vi "与工控机通讯.vi"(10 "values":u16[](array[numeric]), 11 "starting address":u16) -> ()   [LabVIEW 2016, in "斯坦道CODMn.lvlib"]
uses:
  <vilib>/Plasmionique/MB Master/MB_Master_Serial/MB_Master_Serial.lvclass
  C:/Program Files (x86)/National Instruments/LabVIEW 2016/vi.lib/Plasmionique/MB Master/MB_Master/MB_Master.lvclass
  <vilib>/Plasmionique/MB Master/MB Master.lvlib
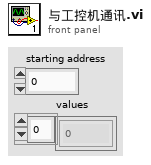
[diagram p1: front panel]
types:
  T1 = cluster{"baud rate (bps)":u32, "stop bits":u16, "parity":u16, "flow control":u16, "timeout":u32, "retries":i32}
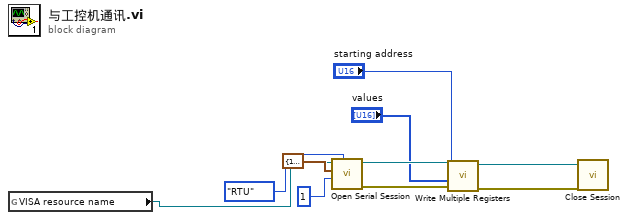
[diagram p0: block diagram]
diagram:
  n1 = global read "COD浓度全局变量.vi" "VISA resource name"() -> (w7:refnum<visa-resource-name>)
  n2 = call <vilib>:"Open Serial Session.vi"("Mode (RTU)"=enum16{"RTU", "ASCII"}."RTU", "Slave ID"=u8 1, "Serial Config"=T1 {"baud rate (bps)"=115200, "stop bits"=10, "parity"=0, "flow control"=0, "timeout"=1000, "retries"=1}, "VISA Resource"=w7) -> ("Error out"=w5:errorcluster, "MB_Serial session"=w6:refnum<class "MB_Master_Serial.lvclass">)  [unwired: 6 in]
  n3 = call <vilib>:"Write Multiple Registers.vi"("error in (no error)"=w5, "values"="values", "starting address"="starting address", "MB session in"=w6) -> ("error out"=w3:errorcluster, "MB session out"=w4:refnum<class "MB_Master_Serial.lvclass">)  [unwired: 6 in]
  n4 = call-dynamic "Close Session.vi"("error in (no error)"=w3, "MB_Serial session"=w4) -> ()  [unwired: 9 in, 1 out]
